vi "Hybrid Distance.vi"(9 "Camera Distance\nfrom Ground (in)":dbl, 10 "Normalized Rect":T2, 11 "Camera Type":T1) -> (2 "Distance (ft)":dbl, 3 "Distance Right (ft)":dbl)   [LabVIEW 2015]
uses:
  Camera Types.ctl
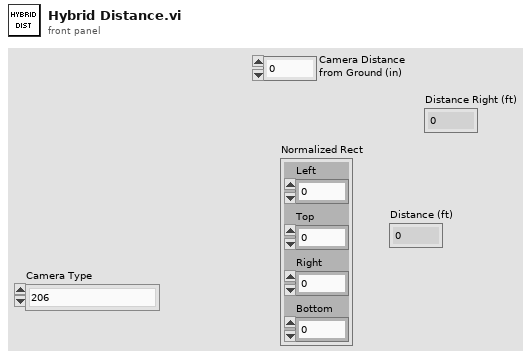
[diagram p1: front panel]
types:
  T1 = typedef "Camera Types.ctl" = enum16{"206", "1011", "1013", "MS HD3000 square", "MS HD3000 640x480"}
  T2 = cluster{"Left":dbl, "Top":dbl, "Right":dbl, "Bottom":dbl}
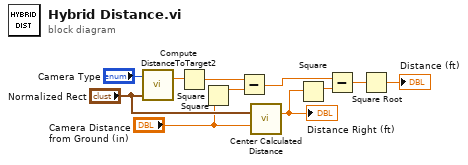
[diagram p0: block diagram]
diagram:
  n1 = call "Compute DistanceToTarget2.vi"("Normalized Rect"="Normalized Rect", "Camera Type"="Camera Type") -> ("Distance (ft)"=w9:dbl)  [unwired: 9 in]
  n2 = Square(x=w9) -> (x^2=w7:dbl)
  n3 = Square(x="Camera Distance\nfrom Ground (in)") -> (x^2=w6:dbl)
  n4 = Subtract(x=w7, y=w6) -> (x-y=w5:dbl)
  n5 = call "Center Calculated Distance.vi"("Camera Distance\nfrom Ground (in)"="Camera Distance\nfrom Ground (in)", "Normalized Rect"="Normalized Rect") -> ("Distance Right (ft)"=w3:dbl)  [unwired: 8 in, 1 out]
  "Distance Right (ft)" <- w3
  n6 = Square(x=w3) -> (x^2=w4:dbl)
  n7 = Subtract(x=w5, y=w4) -> (x-y=w2:dbl)
  n8 = Square Root(x=w2) -> (sqrt(x)=→"Distance (ft)":dbl)
